vi "Example.vi"() -> ()   [LabVIEW 2018]
panel:
  in  "stop":bool
  out "Voltage":dbl
  out "Resistance":dbl
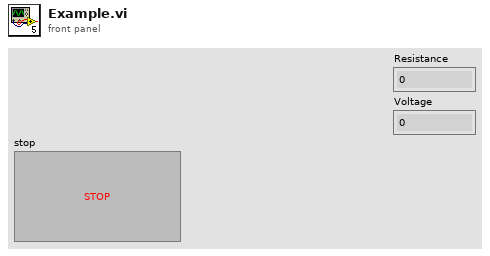
[diagram p1: front panel]
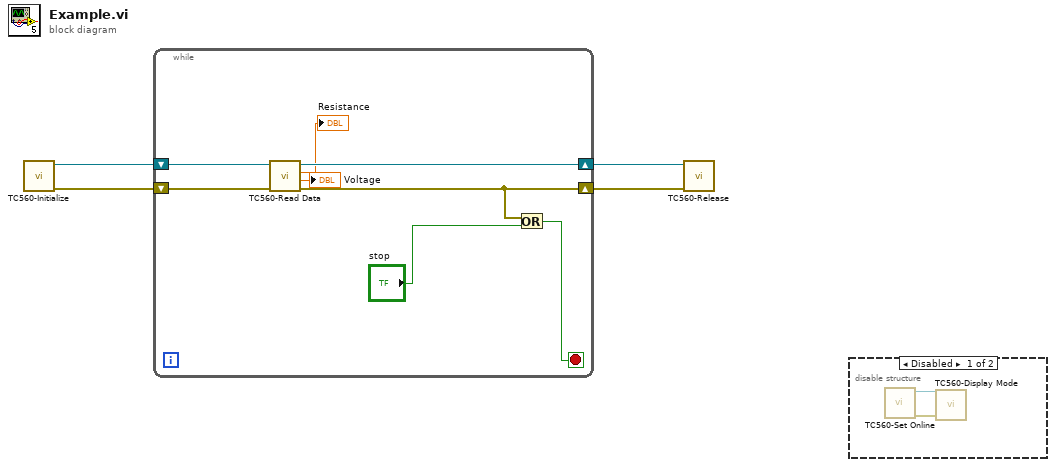
[diagram p0: block diagram]
diagram:
  n1 = call "TC560-Initialize.vi"() -> ("error out"=w2:errorcluster, "VISA Resource Name"=w4:refnum<visa-resource-name>)  [unwired: 10 in]
  n2 = while {
    shift-right: [w11] -> w3
    shift-left: w4 -> [w12]
    shift-right: [w7] -> w1
    shift-left: w2 -> [w10]
    stop <- w5 stop-if-true
    n3 = call "TC560-Read Data.vi"("error in"=w10, "VISA Resource Name In"=w12) -> ("error out"=w7:errorcluster, "Voltage"=→"Voltage":dbl, "Resistance"=→"Resistance":dbl, "VISA Resource Name Out"=w11:refnum<visa-resource-name>)  [unwired: 6 in]
    n4 = Or(x=w7, y="stop") -> (x .or. y?=w5:bool)
  }
  n5 = call "TC560-Release.vi"("error in"=w1, "VISA Resource Name"=w3) -> ()  [unwired: 9 in, 1 out]
  n6 = disable-structure shown="Disabled" {
    frame Disabled {
      n7 = call "TC560-Set Online.vi"() -> ("error out"=w14:errorcluster, "VISA Resource Name Out"=w13:refnum<visa-resource-name>)  [unwired: 9 in, 1 out]
      n8 = call "TC560-Display Mode.vi"("error in"=w14, "VISA Resource Name In"=w13) -> ()  [unwired: 8 in, 2 out]
    }
    frame Enabled {
    }
  }
